vi "파일전송서버.vi"() -> ()   [LabVIEW 2018]
panel:
  in  "파일 리스트":i32(listbox)=-1
  out "Client Connected":bool
  in  "Folder Path":path=path "C:/Users/Public/Pictures/Sample Pictures" caption="저장소 경로"
  out "데이터 출력":string
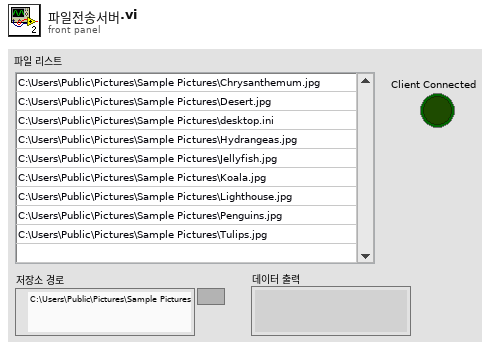
[diagram p1: front panel]
types:
  T1 = enum16{"open", "replace", "create", "open or create", "replace or create", "replace or create with confirmation"}
  T2 = typedef "장난감컨트롤.ctl" = enum16{"대기", "연결됨", "연결종료", "종료", "업데이트", "다운로드"}
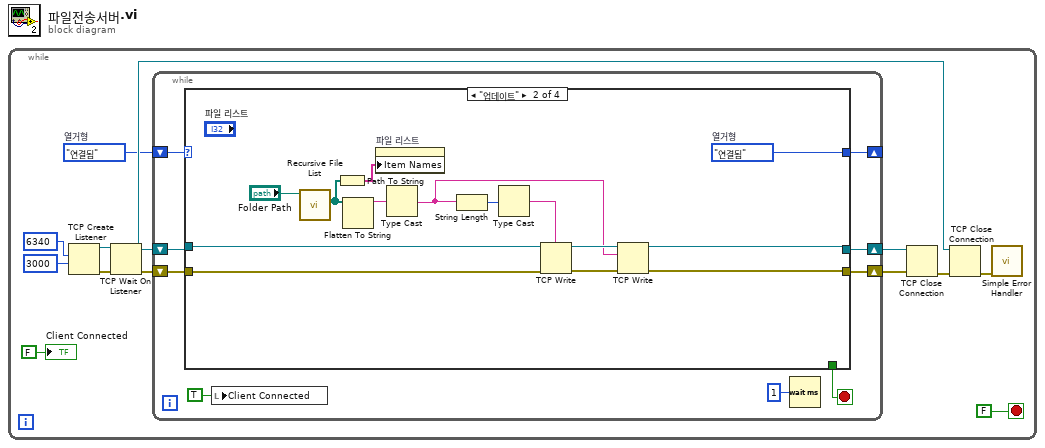
[diagram p0: block diagram]
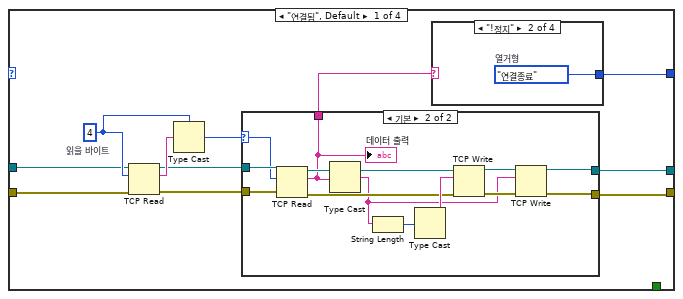
[diagram p2: hidden frame]
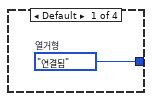
[diagram p3: hidden frame]
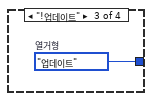
[diagram p4: hidden frame]
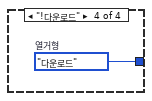
[diagram p5: hidden frame]
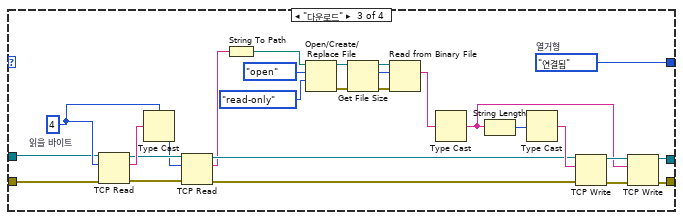
[diagram p7: hidden frame]
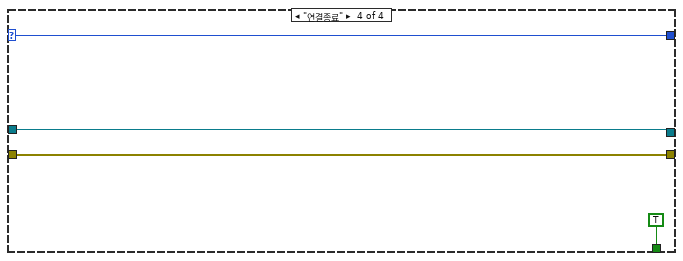
[diagram p8: hidden frame]
diagram:
  n1 = while {
    stop <- FALSE stop-if-true
    w3 = 장난감컨트롤."연결됨"  # 열거형
    n2 = TCP Create Listener(9:3000 ("타임아웃 ms (25000)"), 10:u16 6340 ("포트")) -> (0:w12:errorcluster, 3:w14:refnum<k5>)  [unwired: 3 in, 1 out]
    n3 = TCP Wait On Listener(8:w12, 11:w14) -> (0:w7:errorcluster, 3:w8:refnum<k5>, 4:w5:refnum<k5>)  [unwired: 2 in, 2 out]
    n4 = while {
      shift-right: [w22] -> w6
      shift-left: w7 -> [w23]
      shift-right: [w20] -> w4
      shift-left: w5 -> [w21]
      shift-right: [w18] -> _
      shift-left: w3 -> [w19]
      stop <- w17 stop-if-true
      n5 = case shown="\"업데이트\"" w19 {
        selector: w19 -> [_ _ _ w95]
        tunnel: w23 -> [w31 w59 w78 w96]
        tunnel: [w26 w57 w87 w96] -> w22
        tunnel: w21 -> [w32 w60 w79 w97]
        tunnel: [w27 w58 w88 w97] -> w20
        tunnel: [w24 w67 w94 w95] -> w18
        tunnel: [_ _ _ TRUE] -> w17
        frame "연결됨", Default {
          w33 = 4  # 읽을 바이트
          n6 = TCP Read(connection ID=w32, bytes to read=w33, error in (no error)=w31) -> (connection ID out=w29:refnum<k5>, data out=w34:string, error out=w28:errorcluster)  [unwired: 2 in]
          n7 = Type Cast(type=w33, x=w34) -> (*(type *) &x=w30:i32)
          n8 = case shown="기본" w30 {
            selector: w30 -> [_ w51]
            tunnel: w29 -> [w40 w53]
            tunnel: w28 -> [w39 w52]
            tunnel: [w40 w43] -> w27
            tunnel: [w39 w44] -> w26
            tunnel: [_ w41] -> w25
            frame ..0 {
            }
            frame Default {
              n9 = TCP Read(connection ID=w53, bytes to read=w51, error in (no error)=w52) -> (connection ID out=w49:refnum<k5>, data out=w41:string, error out=w47:errorcluster)  [unwired: 2 in]
              "데이터 출력" <- w41
              n10 = Type Cast(x=w41) -> (*(type *) &x=w42:string)  [unwired: 1 in]
              n11 = String Length(string=w42) -> (length=w50:i32)
              n12 = Type Cast(x=w50) -> (*(type *) &x=w48:string)  [unwired: 1 in]
              n13 = TCP Write(connection ID=w49, data in=w48, error in (no error)=w47) -> (connection ID out=w46:refnum<k5>, error out=w45:errorcluster)  [unwired: 1 in, 1 out]
              n14 = TCP Write(connection ID=w46, data in=w42, error in (no error)=w45) -> (connection ID out=w43:refnum<k5>, error out=w44:errorcluster)  [unwired: 1 in, 1 out]
            }
          }
          n15 = case shown="\"!정지\"" w25 {
            tunnel: [w35 w36 w37 w38] -> w24
            frame Default {
              w35 = 장난감컨트롤."연결됨"  # 열거형
            }
            frame "!정지" {
              w36 = 장난감컨트롤."연결종료"  # 열거형
            }
            frame "!업데이트" {
              w37 = 장난감컨트롤."업데이트"  # 열거형
            }
            frame "!다운로드" {
              w38 = 장난감컨트롤."다운로드"  # 열거형
            }
          }
        }
        frame "업데이트" {
          w67 = 장난감컨트롤."연결됨"  # 열거형
          n16 = call <vilib>:"Recursive File List.vi"("Folder Path"="Folder Path") -> ("All Files in Dir"=w55:path[])  [unwired: 6 in, 4 out]
          n17 = Path To String(path=w55) -> (string=w54:string[])
          n18 = Flatten To String(anything=w55) -> (data string=w61:string)  [unwired: 3 in, 2 out]
          n19 = property on="파일 리스트" class="LstBox (엄격한)"("Item Names"=w54) -> ()  [unwired: 2 in, 2 out]
          n20 = Type Cast(x=w61) -> (*(type *) &x=w64:string)  [unwired: 1 in]
          n21 = String Length(string=w64) -> (length=w63:i32)
          n22 = Type Cast(x=w63) -> (*(type *) &x=w62:string)  [unwired: 1 in]
          n23 = TCP Write(connection ID=w60, data in=w62, error in (no error)=w59) -> (connection ID out=w66:refnum<k5>, error out=w65:errorcluster)  [unwired: 1 in, 1 out]
          n24 = TCP Write(connection ID=w66, data in=w64, error in (no error)=w65) -> (connection ID out=w58:refnum<k5>, error out=w57:errorcluster)  [unwired: 1 in, 1 out]
        }
        frame "다운로드" {
          w80 = 4  # 읽을 바이트
          w94 = 장난감컨트롤."연결됨"  # 열거형
          n25 = TCP Read(connection ID=w79, bytes to read=w80, error in (no error)=w78) -> (connection ID out=w77:refnum<k5>, data out=w81:string, error out=w76:errorcluster)  [unwired: 2 in]
          n26 = Type Cast(type=w80, x=w81) -> (*(type *) &x=w75:i32)
          n27 = TCP Read(connection ID=w77, bytes to read=w75, error in (no error)=w76) -> (connection ID out=w74:refnum<k5>, data out=w72:string, error out=w73:errorcluster)  [unwired: 2 in]
          n28 = String To Path(string=w72) -> (path=w71:path)
          n29 = Open/Create/Replace File(file path (use dialog)=w71, operation (0:open)=T1."open" ("동작(0:open)"), access (0:read/write)=enum16{"read/write", "read-only", "write-only"}."read-only" ("접근(0:읽기/쓰기)")) -> (refnum out=w70:refnum<file>, error out=w85:errorcluster)  [unwired: 3 in, 1 out]
          n30 = Get File Size(file=w70, error in=w85) -> (refnum out=w68:refnum<file>, size (in bytes)=w69:i64, 0:w86:errorcluster)
          n31 = Read from Binary File(8:w86, 10:w69, 11:w68) -> (2:w83:string)  [unwired: 3 in, 3 out]
          n32 = Type Cast(x=w83) -> (*(type *) &x=w91:string)  [unwired: 1 in]
          n33 = String Length(string=w91) -> (length=w90:i32)
          n34 = Type Cast(x=w90) -> (*(type *) &x=w89:string)  [unwired: 1 in]
          n35 = TCP Write(connection ID=w74, data in=w89, error in (no error)=w73) -> (connection ID out=w93:refnum<k5>, error out=w92:errorcluster)  [unwired: 1 in, 1 out]
          n36 = TCP Write(connection ID=w93, data in=w91, error in (no error)=w92) -> (connection ID out=w88:refnum<k5>, error out=w87:errorcluster)  [unwired: 1 in, 1 out]
        }
        frame "연결종료" {
        }
      }
      n37 = local write "Client Connected"(TRUE ("Client Connected")) -> ()
      n38 = Wait (ms)(milliseconds to wait=u32 1 ("대기 시간 (ms)")) -> ()  [unwired: 1 out]
    }
    n39 = TCP Close Connection(connection ID=w4, error in (no error)=w6) -> (error out=w11:errorcluster)  [unwired: 1 in, 1 out]
    n40 = TCP Close Connection(connection ID=w8, error in (no error)=w11) -> (error out=w10:errorcluster)  [unwired: 1 in, 1 out]
    n41 = call <vilib>:"Simple Error Handler.vi"("error in (no error)"=w10) -> ()  [unwired: 4 in, 5 out]
    "Client Connected" <- FALSE ("Client Connected")
  }
